vi "Initialize Population.vi"(6 "# of Genes":u32, 7 "Population Size":u32, 8 "error in":errorcluster, 9 "Gene Type":refnum<class "IGene.lvclass">, 10 "Chromosome Type":refnum<class "IChromosome.lvclass">, 11 "IPopulation in":refnum<class "IPopulation.lvclass">) -> (0 "error out":errorcluster, 3 "IPopulation out":refnum<class "IPopulation.lvclass">)   [LabVIEW 2016, in "IPopulation.lvclass"]
uses:
  IPopulation.lvclass
  IChromosome/IChromosome.lvclass
  IGene/IGene.lvclass
  IPopulation.lvclass/IPopulation.ctl
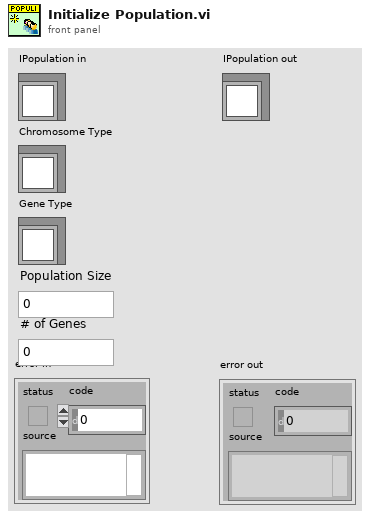
[diagram p1: front panel]
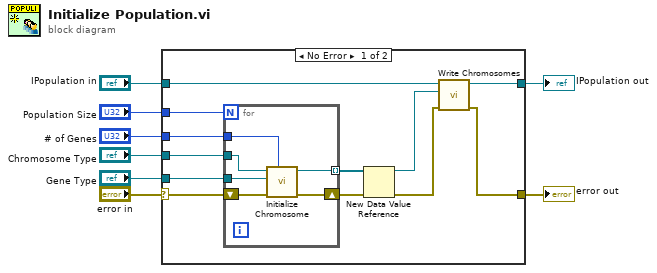
[diagram p0: block diagram]
diagram:
  n1 = case shown="No Error" "error in" {
    selector: "error in" -> [w14 w28]
    tunnel: [w10 w28] -> w7
    tunnel: [w20 w27] -> w5
    tunnel: "IPopulation in" -> [w9 w27]
    tunnel: "Population Size" -> [w15 _]
    tunnel: "Chromosome Type" -> [w18 _]
    tunnel: "# of Genes" -> [w17 _]
    tunnel: "Gene Type" -> [w16 _]
    frame No Error {
      n2 = for {
        N: w15 -> [_]
        tunnel: w18 -> [w26]
        tunnel: w17 -> [w25]
        tunnel: w16 -> [w24]
        shift-right: [w22] -> w12
        shift-left: w14 -> [w23]
        tunnel: [w21] -> w13 mode=indexing
        n3 = call "Initialize Chromosome.vi"("# of Genes"=w25, "error in"=w23, "Gene Type"=w24, "IChromosome in"=w26) -> ("error out"=w22:errorcluster, "IChromosome out"=w21:refnum<class "IChromosome.lvclass">)  [unwired: 6 in]
      }
      n4 = New Data Value Reference(data value=w13, error in=w12) -> (data value reference=w19:refnum<data-value>, error out=w11:errorcluster)
      n5 = call "Write Chromosomes.vi"("error in (no error)"=w11, "Chromosomes"=w19, "IPopulation in"=w9) -> ("error out"=w10:errorcluster, "IPopulation out"=w20:refnum<class "IPopulation.lvclass">)  [unwired: 7 in]
    }
    frame Error {
    }
  }
  "error out" <- w7
  "IPopulation out" <- w5
